vi "test tbm module metadata.vi"() -> ()   [LabVIEW 2013, in "TBM Tests.lvlib"]
uses:
  TBM Tests.lvlib
  root configuration/TBM configuration.lvclass
panel:
  out "overwriteok":bool
  out "setgetok":bool
  out "deletedok":bool
  out "ook":errorcluster
  out "error 538311":errorcluster
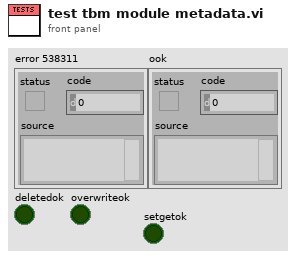
[diagram p1: front panel]
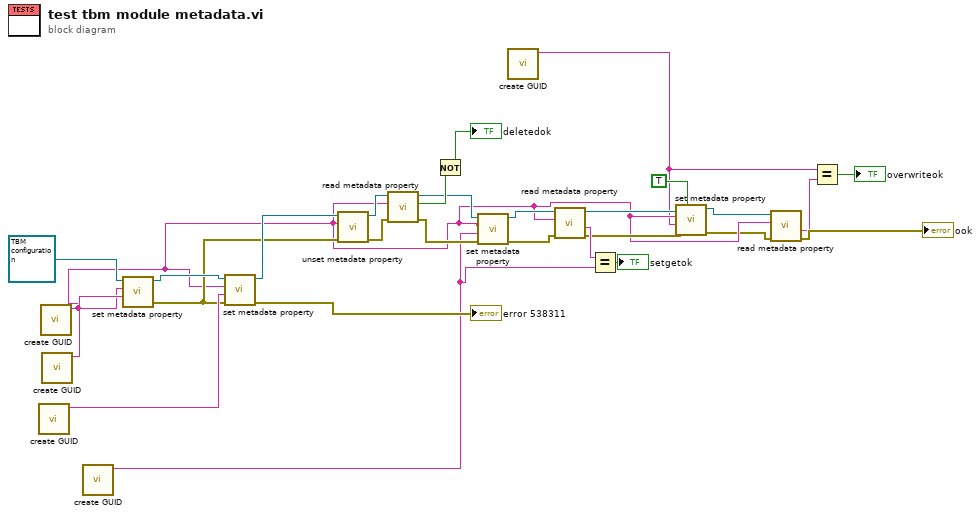
[diagram p0: block diagram]
diagram:
  n1 = call "create GUID.vi"() -> ("uuid"=w24:string)  [unwired: 11 in]
  n2 = call "create GUID.vi"() -> ("uuid"=w6:string)  [unwired: 11 in]
  n3 = call "create GUID.vi"() -> ("uuid"=w25:string)  [unwired: 11 in]
  n4 = call "create GUID.vi"() -> ("uuid"=w13:string)  [unwired: 11 in]
  n5 = call "set metadata property.vi"("value"=w25, "key"=w6, "configuration in"=refnum<class "TBM configuration.lvclass"> refnum ("configuration")) -> ("error out"=w22:errorcluster, "configuration out"=w27:refnum<class "TBM configuration.lvclass">)  [unwired: 7 in]
  n6 = call "set metadata property.vi"("error in"=w22, "value"=w24, "key"=w6, "configuration in"=w27) -> ("error out"=→"error 538311":errorcluster, "configuration out"=w23:refnum<class "TBM configuration.lvclass">)  [unwired: 6 in]
  n7 = call "unset metadata property.vi"("error in"=w22, "key"=w6, "configuration in"=w23) -> ("error out"=w21:errorcluster, "configuration out"=w20:refnum<class "TBM configuration.lvclass">)  [unwired: 7 in]
  n8 = call "read metadata property.vi"("error in"=w21, "key"=w6, "configuration in"=w20) -> ("error out"=w18:errorcluster, "found"=w19:bool, "configuration out"=w17:refnum<class "TBM configuration.lvclass">)  [unwired: 5 in, 1 out]
  n9 = Not(x=w19) -> (.not. x?=→"deletedok":bool)
  n10 = call "set metadata property.vi"("error in"=w18, "value"=w13, "key"=w6, "configuration in"=w17) -> ("error out"=w16:errorcluster, "configuration out"=w15:refnum<class "TBM configuration.lvclass">)  [unwired: 6 in]
  n11 = call "create GUID.vi"() -> ("uuid"=w2:string)  [unwired: 11 in]
  n12 = call "read metadata property.vi"("error in"=w16, "key"=w6, "configuration in"=w15) -> ("error out"=w10:errorcluster, "value"=w14:string, "configuration out"=w9:refnum<class "TBM configuration.lvclass">)  [unwired: 5 in, 1 out]
  n13 = Equal?(x=w14, y=w13) -> (x = y?=→"setgetok":bool)
  n14 = call "set metadata property.vi"("overwrite?"=TRUE, "error in"=w10, "value"=w2, "key"=w6, "configuration in"=w9) -> ("error out"=w5:errorcluster, "configuration out"=w7:refnum<class "TBM configuration.lvclass">)  [unwired: 5 in]
  n15 = call "read metadata property.vi"("error in"=w5, "key"=w6, "configuration in"=w7) -> ("error out"=→"ook":errorcluster, "value"=w3:string)  [unwired: 5 in, 2 out]
  n16 = Equal?(x=w2, y=w3) -> (x = y?=→"overwriteok":bool)
